vi "Intake Controller.vi"(8 "error in":errorcluster) -> ()   [LabVIEW 2017]
doc: "This VI executes continuously carrying out the current operation and responding to updates or new operations. It will often contain the timing or control code that is difficult to place directly in TeleOp. This VI generally opens all sensors and motors and isolates the rest of the robot code from knowing how the operations are carried out."
uses:
  <vilib>/Rock Robotics/WPI/Framework/Completion Status.ctl
  Intake Setpoints.ctl
  Intake Operations.ctl
  <vilib>/Rock Robotics/WPI/SafetyOutput/WPI_SafetyOutputConfigMenu.ctl
  Intake Motor Settings.ctl
  <vilib>/Rock Robotics/SystemInterfaces/DIO/FPGA_DIOPWMChannel.ctl
  <vilib>/Rock Robotics/Network Tables/NT Write Boolean.vi
panel:
  out "Setpoints":T1(graph)
  in  "Interactive Values":T2
  out "Current\nCmd":string
  in  "Buttons":cluster{"Execute Cmd":bool, "Abort Cmd":bool}
  out "Command Timing":cluster{"Start Time (ms)":u32, "Iterations":i32}
  out "Status":T4
  # "Tip: It may be helpful to observe inputs and sensor values.\nYou may also want to display tuning or debugging controls."
  # "Interactive Command: You may fill in the settings for a command\nand schedule it with the Execute button. You can observe and abort\nany command while fine tuning the code for the controller."
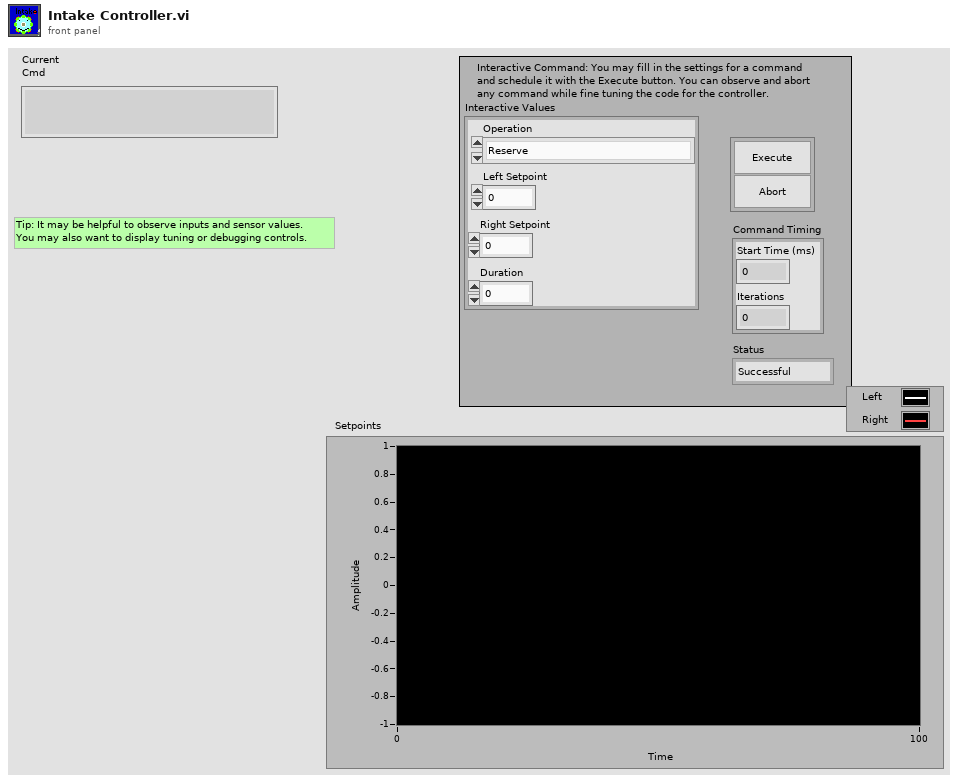
[diagram p1: front panel]
types:
  T1 = cluster{"Left Setpoint":dbl, "Right Setpoint":dbl}
  T2 = typedef "Intake Setpoints.ctl" = cluster{"Operation":T3, "Left Setpoint":dbl, "Right Setpoint":dbl, "Duration":dbl}
  T3 = typedef "Intake Operations.ctl" = enum16{"Reserve", "Read Current", "Immediate", "Intake with Duration"}
  T4 = typedef "Completion Status.ctl" = enum16{"Successful", "Aborted", "Incomplete"}
  T5 = typedef "Intake Motor Settings.ctl" = cluster{"Left Motor":cluster{"Inversion":bool, "PWM Channel":T6}, "Right Motor":cluster{"Inversion":bool, "PWM Channel":T6}}
  T6 = typedef "FPGA_DIOPWMChannel.ctl" = enum8{"PWM 0", "PWM 1", "PWM 2", "PWM 3", "PWM 4", "PWM 5", "PWM 6", "PWM 7", "PWM 8", "PWM 9", "PWM MXP 0", "PWM MXP 1", "PWM MXP 2", "PWM MXP 3", "PWM MXP 4", "PWM MXP 5", "PWM MXP 6", "PWM MXP 7", "PWM MXP 8", "PWM MXP 9", "Invalid"}
  T7 = typedef "WPI_SafetyOutputConfigMenu.ctl" = enum16{"Enable", "Disable"}
  T8 = typedef "WPI_RobotDriveDevRef.ctl" = cluster{"DevStatus":errorcluster, "Motors[]":T9[], "Square Inputs":bool, "Max Output":dbl}
  T9 = typedef "WPI_MotorControlDeviceRef.ctl" = cluster{"DeviceStatus":errorcluster, "Type":T10, "PWM":cluster{"PWM Channel":T6, "DeadBand":T11}, "CAN":cluster{"Device Number":u8, "SetOutput VI Ref":variant, "GetOutput VI Ref":variant, "Enable VI Ref":variant, "Disable VI Ref":variant, "Data":variant}, "Invert":bool, "DIO PWM":cluster{"PWM \"Enable\" Channel":T6, "DIOChannel":T12, "PWM Rate":dbl}}
  T10 = typedef "WPI_MotorControlType.ctl" = enum16{"PWM", "CAN", "DIO PWM"}
  T11 = typedef "WPI_PWMDeadband.ctl" = cluster{"Name":string, "maxPositivePwm":i32, "minPositivePwm":i32, "centerPwm":i32, "maxNegativePwm":i32, "minNegativePwm":i32, "angularRange":u16}
  T12 = typedef "FPGA_DIOChannel.ctl" = enum8{"DIO 0", "DIO 1", "DIO 2", "DIO 3", "DIO 4", "DIO 5", "DIO 6", "DIO 7", "DIO 8", "DIO 9", "DIO MXP 0", "DIO MXP 1", "DIO MXP 2", "DIO MXP 3", "DIO MXP 4", "DIO MXP 5", "DIO MXP 6", "DIO MXP 7", "DIO MXP 8", "DIO MXP 9", "DIO MXP 10", "DIO MXP 11", "DIO MXP 12", "DIO MXP 13", "DIO MXP 14", "DIO MXP 15", "SPI Port CS1", "SPI Port CS2", "SPI Port CS3", "SPI Port MISO", "SPI Port MOSI", "Invalid"}
  T13 = typedef "Command Status Info.ctl" = cluster{"Name":string, "Status":T4, "notifier out":T14}
  T14 = typedef "Completion Notifier.ctl" = refnum<notifier>
  T15 = cluster{"Current Command":T2, "Command Timing":cluster{"Start Time (ms)":u32, "Iterations":i32}, "Command Arguments":cluster{"Command Info":T13, "Description":string, "Default Command":T2, "queue out":refnum<queue>, "Subsystem Name":string}}
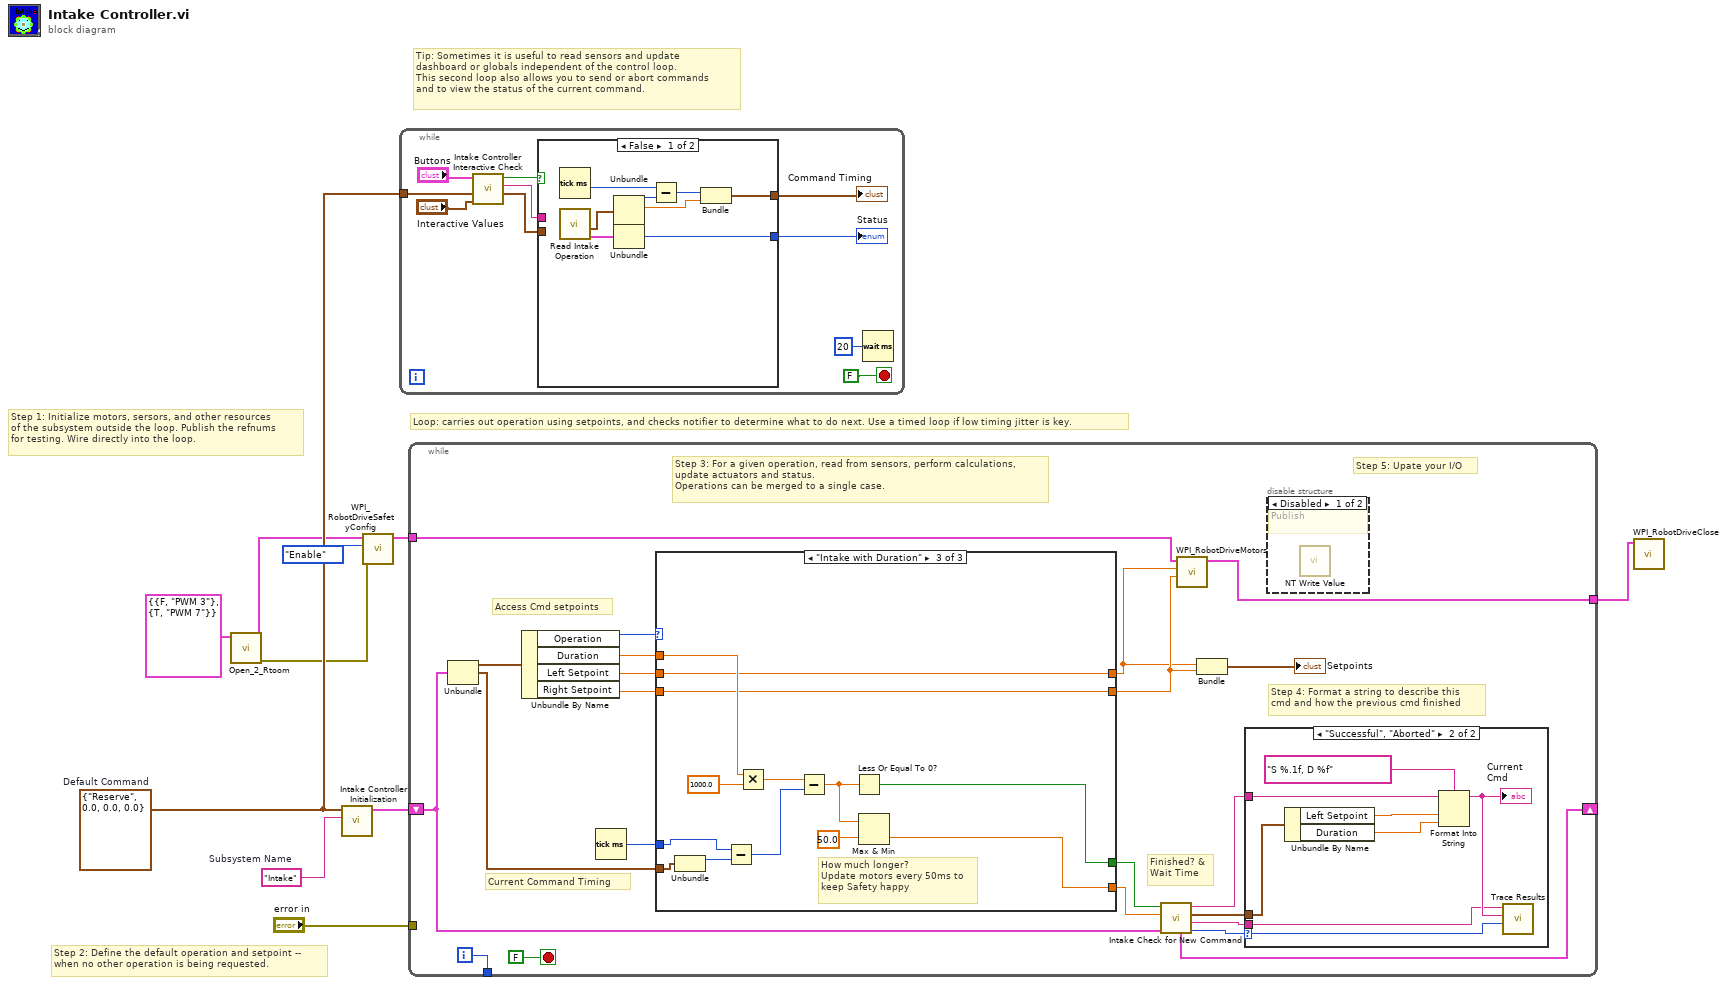
[diagram p0: block diagram]
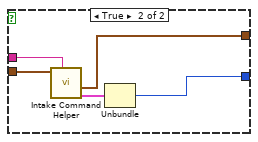
[diagram p2: hidden frame]
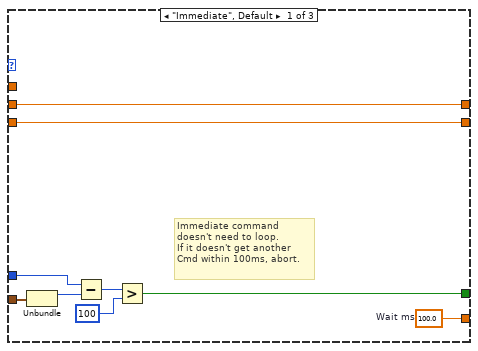
[diagram p5: hidden frame]
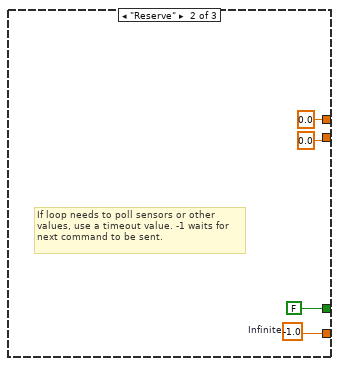
[diagram p6: hidden frame]
diagram:
  w7 = T2 {"Operation"=enum."Reserve", "Left Setpoint"=0.0, "Right Setpoint"=0.0, "Duration"=0.0}  # Default Command
  w8 = "Intake"  # Subsystem Name
  # "Tip: Sometimes it is useful to read sensors and update\ndashboard or globals independent of the control loop.\nThis second loop also allows you to send or abort commands\nand to view the status of the current command."
  # "Step 2: Define the default operation and setpoint --\nwhen no other operation is being requested."
  # "Step 1: Initialize motors, sersors, and other resources\nof the subsystem outside the loop. Publish the refnums\nfor testing. Wire directly into the loop."
  # "Loop: carries out operation using setpoints, and checks notifier to determine what to do next. Use a timed loop if low timing jitter is key."
  n1 = call "Open_2_Rtoom.vi"("Motor Settings"=T5 {"Left Motor"={"Inversion"=FALSE, "PWM Channel"=enum."PWM 3"}, "Right Motor"={"Inversion"=TRUE, "PWM Channel"=enum."PWM 7"}}) -> ("error out"=w5:errorcluster, "RobotDriveDevRef"=w6:T8)  [unwired: 8 in]
  n2 = call "Intake Controller Initialization.vi"("Subsystem Name"=w8, "Default Command"=w7) -> ("Current Command"=w9:T15)  [unwired: 9 in]
  n3 = call <vilib>:"WPI_RobotDriveSafetyConfig.vi"("error in (no error)"=w5, "mode"=WPI_SafetyOutputConfigMenu."Enable", "RobotDriveDevRef"=w6) -> ("RobotDriveDevRef"=w4:T8)  [unwired: 7 in, 1 out]
  n4 = while {
    tunnel: w7 -> [w17]
    stop <- FALSE stop-if-true
    n5 = call "Intake Controller Interactive Check.vi"("Interactive Command in"="Interactive Values", "Default Command"=w17, "Buttons"="Buttons") -> ("Interactive Command out"=w15:T2, "Trace String"=w16:string, "Schedule"=w11:bool)  [unwired: 6 in]
    n6 = case shown="False" w11 {
      tunnel: [w28 w33] -> w14
      tunnel: w15 -> [_ w31]
      tunnel: [w24 w29] -> w13
      tunnel: w16 -> [_ w32]
      frame False {
        n7 = Tick Count (ms)() -> (millisecond timer value=w23:u32)
        n8 = call "Read Intake Operation.vi"() -> ("Command Info"=w21:T13, "SubSystem Data"=w22:T2)  [unwired: 9 in, 1 out]
        n9 = Unbundle(w22) -> ("Operation"=w27:T3, "Left Setpoint"=w25:dbl)  [unwired: 2 out]
        n10 = Unbundle(w21) -> ("Status"=w28:T4)  [unwired: 2 out]
        n11 = Subtract(x=w23, y=w27) -> (x-y=w26:u32)
        n12 = Bundle(w26, "Left Setpoint"=w25) -> (w24:cluster{u32, "Left Setpoint":dbl})  [unwired: 1 in]
      }
      frame True {
        n13 = call "Intake Command Helper.vi"("Description"=w32, "SubSystem Data"=w31) -> ("Command Info Out"=w30:T13, "Command Timing"=w29:cluster{"Start Time (ms)":u32, "Iterations":i32})  [unwired: 7 in, 1 out]
        n14 = Unbundle(w30) -> ("Status"=w33:T4)  [unwired: 2 out]
      }
    }
    "Status" <- w14
    "Command Timing" <- w13
    n15 = Wait (ms)(milliseconds to wait=u32 20) -> ()  [unwired: 1 out]
  }
  n16 = while {
    shift-right: [w48] -> _
    shift-left: w9 -> [w41]
    tunnel: [w54] -> _
    tunnel: "error in" -> [_]
    tunnel: w4 -> [w36]
    tunnel: [w35] -> w3
    i -> [w54]
    stop <- FALSE stop-if-true
    # "Step 5: Upate your I/O"
    # "Step 4: Format a string to describe this\ncmd and how the previous cmd finished"
    # "Current Command Timing"
    # "Access Cmd setpoints"
    # "Finished? &\nWait Time"
    # "Step 3: For a given operation, read from sensors, perform calculations,\nupdate actuators and status.\nOperations can be merged to a single case."
    n17 = Unbundle(w41) -> ("Current Command"=w53:T2, "Command Timing"=w50:cluster{"Start Time (ms)":u32, "Iterations":i32})  [unwired: 1 out]
    n18 = Unbundle By Name(w53) -> ("Operation"=w52:T3, "Duration"=w39:dbl, "Left Setpoint"=w49:dbl, "Right Setpoint"=w40:dbl)
    n19 = Tick Count (ms)() -> (millisecond timer value=w51:u32)
    n20 = case shown="\"Intake with Duration\"" w52 {
      tunnel: [w72 w76 w82] -> w46
      tunnel: [w66 FALSE ("ignore previous (F)") w83] -> w47
      tunnel: w50 -> [w68 _ w81]
      tunnel: w51 -> [w67 _ w80]
      tunnel: w49 -> [w65 _ w78]
      tunnel: w40 -> [w64 _ w77]
      tunnel: w39 -> [_ _ w79]
      tunnel: [w65 0.0 ("Left Setpoint") w78] -> w37
      tunnel: [w64 0.0 ("Right Setpoint") w77] -> w38
      frame "Immediate", Default {
        w72 = 100.0  # Wait ms
        # "Immediate command\ndoesn't need to loop.\nIf it doesn't get another\nCmd within 100ms, abort."
        n21 = Unbundle(w68) -> ("Start Time (ms)"=w71:u32)  [unwired: 1 out]
        n22 = Subtract(x=w67, y=w71) -> (x-y=w70:u32)
        n23 = Greater?(x=w70, y=u8 100 ("Left Motor")) -> (0:w66:bool)
      }
      frame "Reserve" {
        w76 = -1.0  # Infinite
        # "If loop needs to poll sensors or other\nvalues, use a timeout value. -1 waits for\nnext command to be sent."
      }
      frame "Intake with Duration" {
        # "How much longer?\nUpdate motors every 50ms to\nkeep Safety happy"
        n24 = Unbundle(w81) -> ("Start Time (ms)"=w86:u32)  [unwired: 1 out]
        n25 = Subtract(x=w80, y=w86) -> (x-y=w89:u32)
        n26 = Multiply(x=w79, y=1000.0) -> (x*y=w88:dbl)
        n27 = Subtract(x=w88, y=w89) -> (x-y=w85:dbl)
        n28 = Less Or Equal To 0?(x=w85) -> (x <= 0?=w83:bool)
        n29 = Max & Min(x=w85, y=50.0) -> (min(x,y)=w82:dbl)  [unwired: 1 out]
      }
    }
    n30 = call "Intake Check for New Command.vi"("Current Command"=w41, "Wait time (ms)"=w46, "Finished?"=w47) -> ("Completion"=w42:T4, "Subsystem Name"=w43:string, "Current Command"=w44:T2, "Initial Trace String"=w45:string, "NextCommand"=w48:T15)  [unwired: 4 in]
    n31 = call <vilib>:"WPI_RobotDriveMotors.vi"("RightSpeed"=w38, "LeftSpeed"=w37, "RobotDriveDevRef"=w36) -> ("RobotDriveDevRef"=w35:T8)  [unwired: 6 in, 2 out]
    n32 = Bundle("Left Setpoint"=w37, "Right Setpoint"=w38) -> (→"Setpoints":T1)  [unwired: 1 in]
    n33 = case shown="\"Successful\", \"Aborted\"" w42 {
      selector: w42 -> [_ w63]
      tunnel: w45 -> [_ w59]
      tunnel: w44 -> [_ w60]
      tunnel: w43 -> [_ w56]
      frame "Incomplete", Default {
        # "Continuing current command"
      }
      frame "Successful", "Aborted" {
        # "Report and setup for next command"
        n34 = Unbundle By Name(w60) -> ("Left Setpoint"=w62:dbl, "Duration"=w57:dbl)
        n35 = Format Into String(format string="S %.1f, D %f", initial string=w59, w62, w57) -> (resulting string=w58:string)  [unwired: 1 in, 1 out]
        "Current\nCmd" <- w58
        n36 = call <vilib>:"Trace Results.vi"("Status of previous command"=w63, "Description"=w58, "Subsystem"=w56) -> ()  [unwired: 9 in]
      }
    }
    n37 = disable-structure shown="Disabled" {
      frame Disabled {
        # "Publish"
        n38 = call-poly <vilib>:"NT Write Value.vi"() -> ()  [unwired: 11 in, 1 out]
      }
      frame Enabled {
      }
    }
  }
  n39 = call <vilib>:"WPI_RobotDriveClose.vi"("RobotDriveDevRef"=w3) -> ()  [unwired: 10 in, 1 out]
